vi "Main FPGA 5-axis with 1AxisLimitU8.vi"() -> ()   [LabVIEW 2013]
uses:
  <vilib>/Motion/MotorControl/_s/nism.interpretControlRegister.stateTransition.ctl
  <vilib>/Platform/TimedLoop/XDataNode/timing_clust.ctl
  <vilib>/Platform/TimedLoop/XDataNode/nitl_modes.ctl
  <vilib>/Platform/TimedLoop/XDataNode/wakeup.ctl
  <vilib>/Motion/MotorControl/_s/nism.digitalInputs.portA.ctl
  <vilib>/rvi/Emulation/niFpgaSctlEmulationGetInTimedLoop.vi
  <vilib>/rvi/Emulation/niFpgaEmulationReportErrorSimple.vi
  <vilib>/rvi/Emulation/niFpgaGetClockAttributes.vi
  <vilib>/rvi/Emulation/niFpgaCriticalErrorInLSC.vi
  Global FPGA.vi
  <vilib>/rvi/eio/common/nirviEmuTemplateMethod_errors.vi
  <vilib>/Motion/SoftMotion/Synchronization/nism.rioScan.generateSyncScan.vi
  <vilib>/rvi/Emulation/niFpgaProcessEmulError.vi
  <vilib>/Motion/MotorControl/_s/nism.interpretControlRegister.indexed.vi
  <vilib>/Motion/MotorControl/_s/nism.generateStatusRegister.indexed.vi
  <vilib>/Motion/MotorControl/_s/nism.mdo.read.positionLoopSyncData.vi
  <vilib>/Motion/MotorControl/_s/nism.mdo.read.splineData.vi
  <vilib>/Motion/MotorControl/_s/nism.splineInterpolation.fxp.3.index.vi
  <vilib>/Motion/MotorControl/_s/nism.mdo.handler.indexed.vi
  <vilib>/Motion/MotorControl/_s/nism.interpretDIOControl.portA.single.2.vi
  <vilib>/Motion/MotorControl/_s/nism.generateDIOStatus.portA.single.vi
  <vilib>/Platform/TimedLoop/XDataNode/XDataNode.xnode
  <vilib>/eio/EIONode/EIONode.xnode
  <vilib>/Motion/MotorControl/NI_SoftMotion_MotorControlIP.lvlib
  <vilib>/Platform/TimedLoop/XDataNode/XDNodeRunTimeDep.lvlib
  <vilib>/Motion/SoftMotion/Synchronization/NI_SoftMotion_Synchronization.lvlib
panel:
  in  "Axi1 1 DI":u8
  out "Axis Positions":fxp<+/-,64,32>[](array[numeric])
  in  "STEP or CW? (T=STEP)":bool
  out "Drive Enable":bool[](array[boolean])
  in  "Enable Watchdog":bool
  in  "Pet Watchdog":bool
  in  "Watchdog Timeout Period (ticks)":u64=40000000 format="%.0p"
  out "Watchdog Timed Out?":bool
  out "Time Since Last Pet":u64
  in  "Enable value":bool
  in  "Drive Enable override?":bool
  out "State":T1=enum."Start --> Initializing" caption="state transition"
  in  "Sync Value":bool
  in  "Sync Enable override?":bool
  in  "Invert direction?":bool
  out "Sync is Fault":bool
  out "Sync is Locked":bool
  in  "minimum pulse":u16=40
  # "Synchronization Loop"
  # "Control Status Loop"
  # "Notes: \n1. This VI provides the communication interface between the NI SoftMotion Engine and the LabVIEW FPGA Module. You must compile this VI for a specific FPGA target before use. After compiling, run the VI before running any of the Express VI examples. For information on moving this example to another FPGA target, refer to ni.com/info and enter info code fpgaex.\n\n2. Only use the Reset Axis button if you are unable to communicate with the axis by any other means. This button resets the device state machine and other VIs to a known state. After resetting the axis, switch the NI Scan Engine from Active Mode to Configuration Mode, then back to Active Mode, before attempting to enable the axis."
  # "(These two buttons \nare for testing\npurposes.)"
  # "(These two buttons \nare for testing\npurposes.)"
  # "Step/Direction Loop"
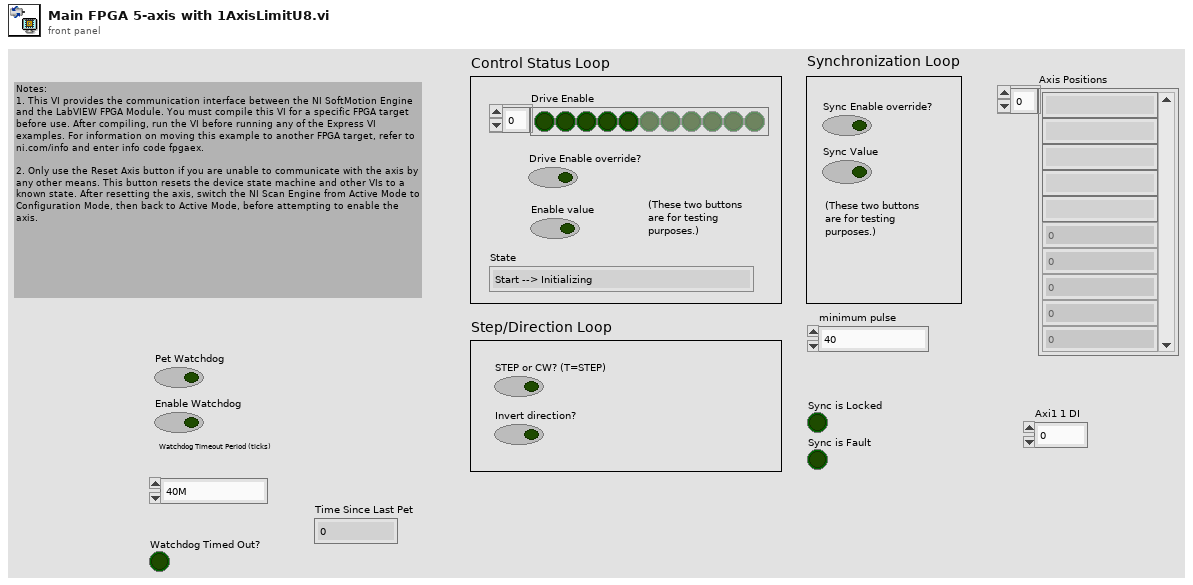
[diagram p1: front panel]
types:
  T1 = typedef "NI_SoftMotion_MotorControlIP.lvlib/nism.interpretControlRegister.stateTransition.ctl" = enum8{"Invalid", "Start --> Initializing", "Initializing --> Disabled", "Disabled --> Ready To Switch On", "Ready To Switch On --> Switched On", "Ready To Switch On --> Disable", "Switched On --> Operation Enable", "Switched On --> Ready To Switch On", "Switched On --> Disabled", "Operation Enable --> Switched On", "Operation Enable --> Ready To Switch On", "Operation Enable --> Disabled", "Fault --> Disabled", "Any --> Fault", "None"}
  T2 = typedef "NI_SoftMotion_MotorControlIP.lvlib/nism.mdo.splineData.ctl" = cluster{"spline type":T3, "traj per/spline per":u16, "spline per/traj per":fxp<+,32,0>}
  T3 = typedef "nism.splineInterpolation.type.ctl" = u16
  T4 = typedef "NI_SoftMotion_Synchronization.lvlib/nism.softmotionScan.timerConfig.ctl" = cluster{"Target Period (clocks)":u16, "Host Period / Target Period":u16}
  T5 = typedef "XDNodeRunTimeDep.lvlib/timing_clust.ctl" = cluster{"Expected End [f-1]":u64, "Actual End [f-1]":u64, "Finished Late? [f-1]":bool, "Expected End [i-1]":u64, "Actual End [i-1]":u64, "Finished Late? [i-1]":bool, "Expected Start [i]":u64, "Actual Start [i]":u64, "Expected Start [f]":u64, "Actual Start [f]":u64, "Source Name":string, "Structure Name":string, "Period":i64, "Deadline":i64, "Offset":i64, "Start":i64, "Priority":i32, "Timeout":i32, "Mode":T6, "Wakeup Reason":T7, "Error":errorcluster, "Source Type":string, "Secondary Source Type":string, "Global End Time":u64, "Global Start Time":u64, "Frame Duration":u64, "Iteration Duration":u64, "Assigned CPU":i32, "I/O Scan Engine Mode":u32}
  T6 = typedef "XDNodeRunTimeDep.lvlib/nitl_modes.ctl" = enum32{"No Change", "Process missed periods, maintain original phase", "Discard missed periods, maintain original phase", "Process missed periods, ignore original phase", "Discard missed periods, ignore original phase"}
  T7 = typedef "XDNodeRunTimeDep.lvlib/wakeup.ctl" = enum32{"Normal", "Aborted", "Asynchronous wakeup", "Timing source error", "Timed loop error", "Timeout"}
  T8 = typedef "NI_SoftMotion_Synchronization.lvlib/nism.softmotionScan.timerControl.ctl" = cluster{"SM Scan":bool, "SM Scan Count":u32, "SM Scan Enabled":bool}
  T9 = typedef "NI_SoftMotion_MotorControlIP.lvlib/nism.digitalInputs.portA.ctl" = cluster{"reverse limit":bool, "forward limit":bool, "home switch":bool, "digital input 0":bool, "digital input 1":bool, "digital input 2":bool, "digital input 3":bool}
  T10 = typedef "NI_SoftMotion_MotorControlIP.lvlib/nism.dio.portA.config.2.ctl" = cluster{"digital filter (us)":u16[], "safe state":enum16{"Low", "High", "No Change"}[]}
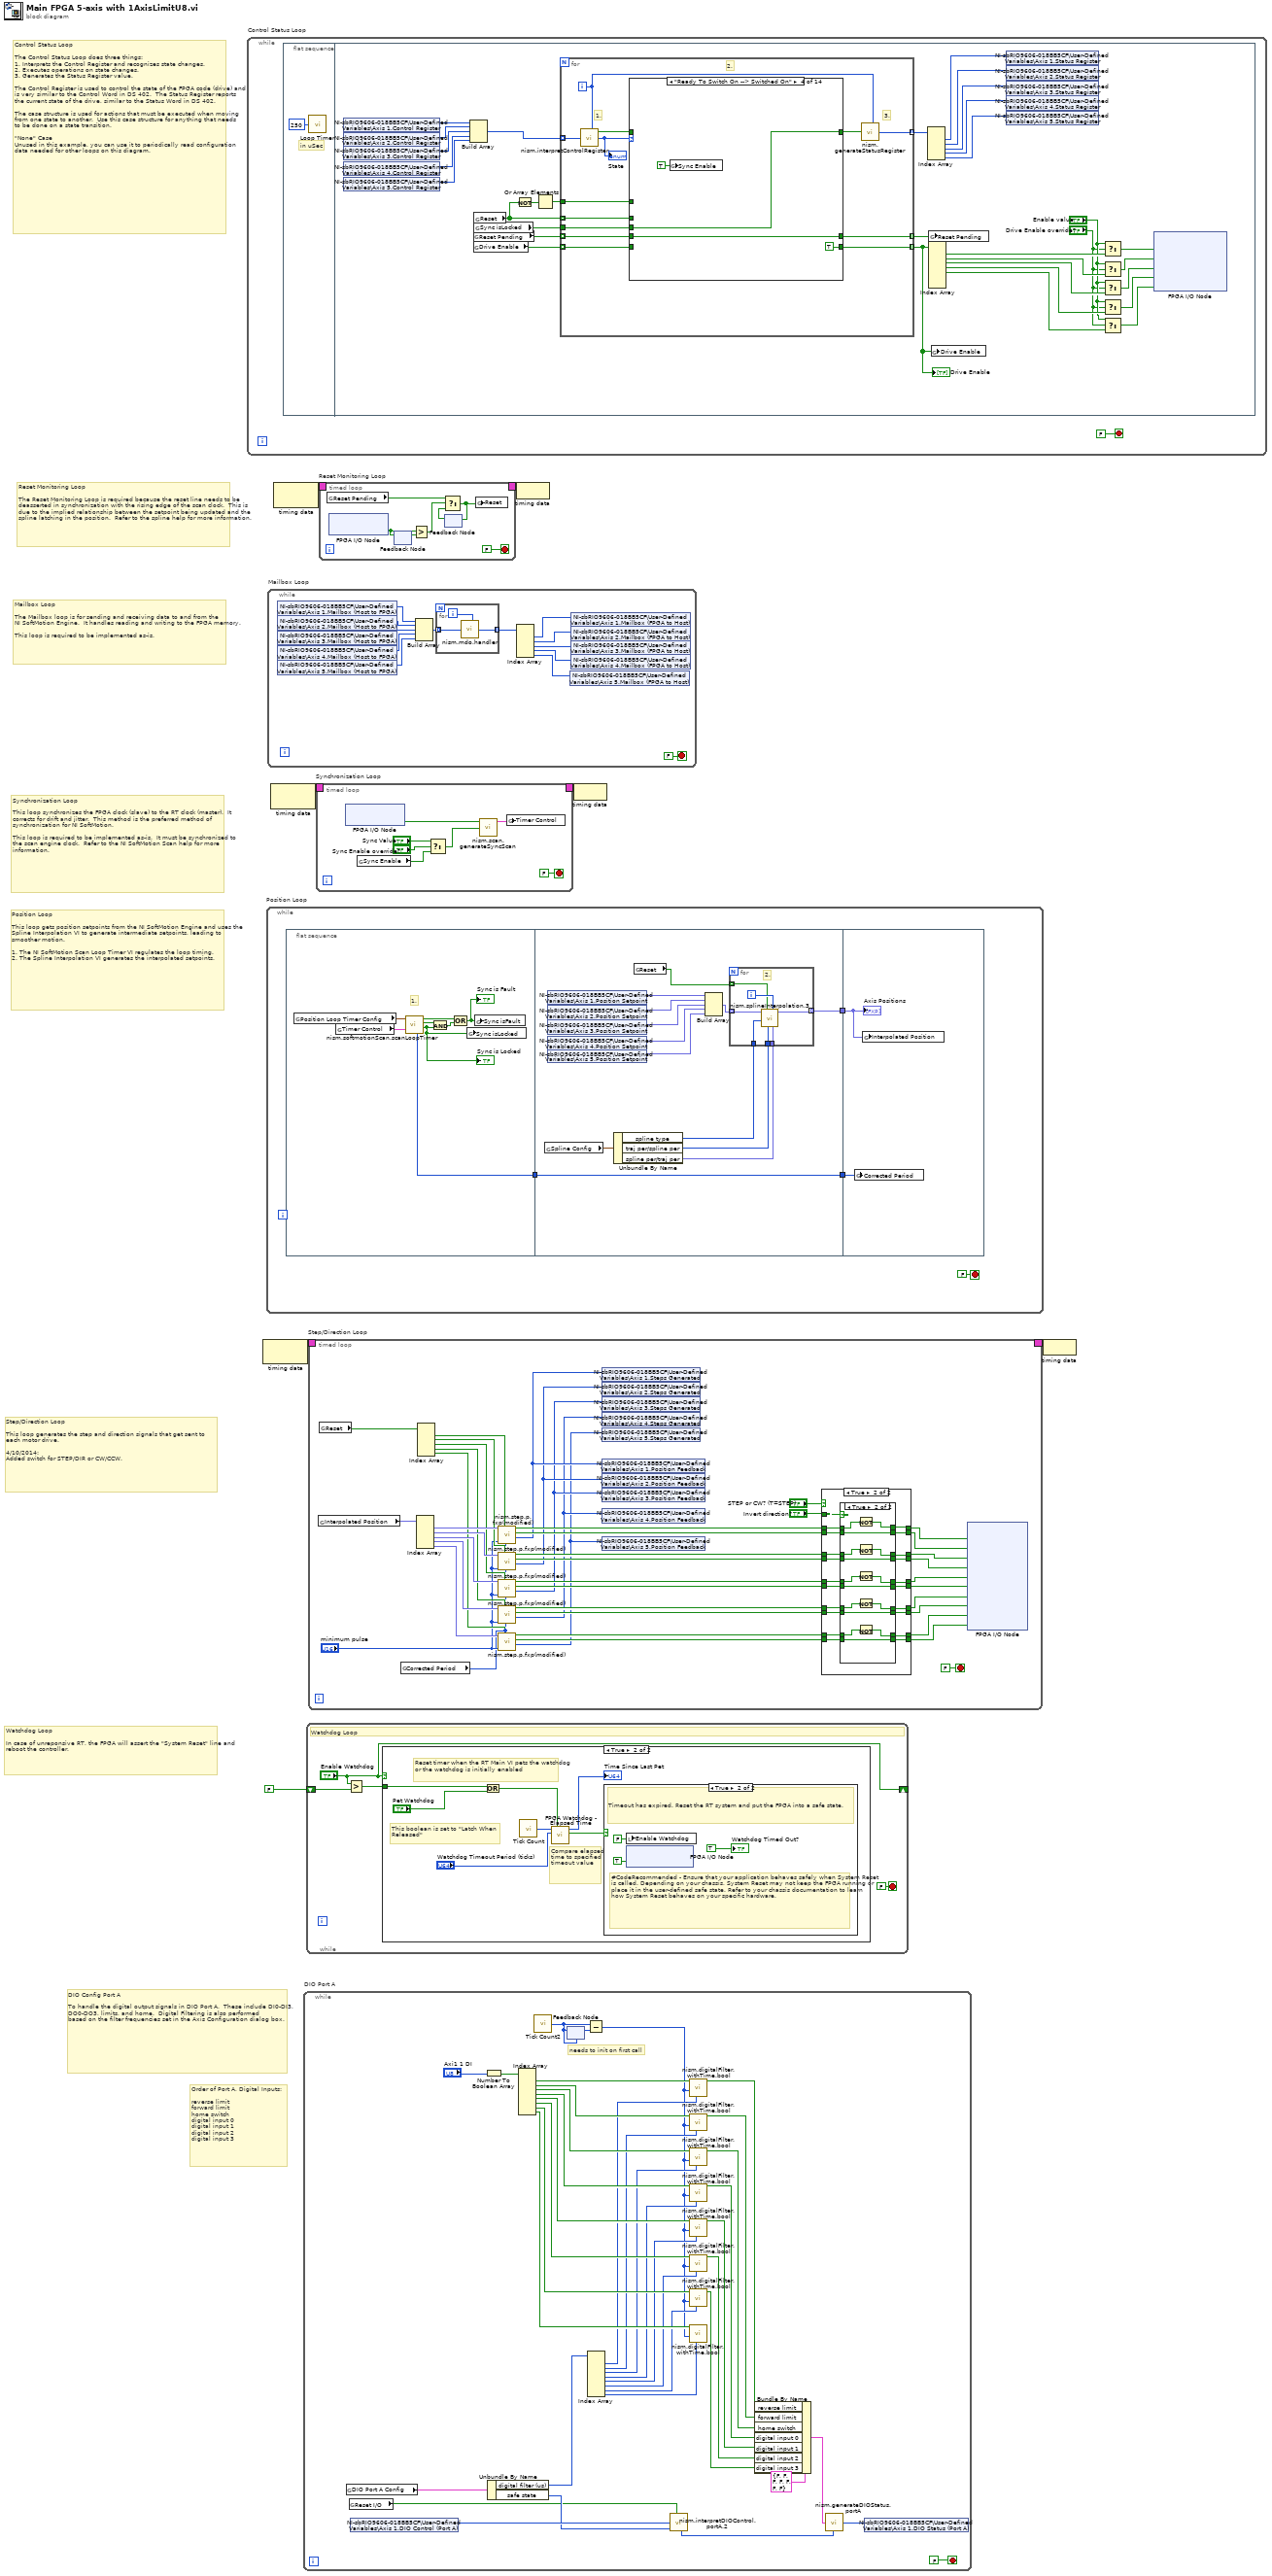
[diagram p0: block diagram]
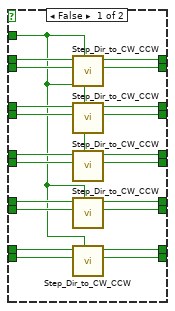
[diagram p4: hidden frame]
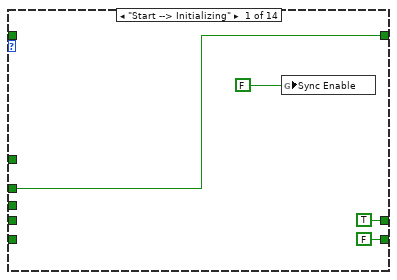
[diagram p6: hidden frame]
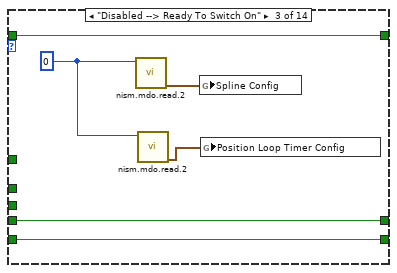
[diagram p8: hidden frame]
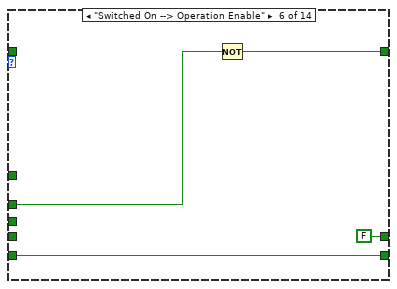
[diagram p10: hidden frame]
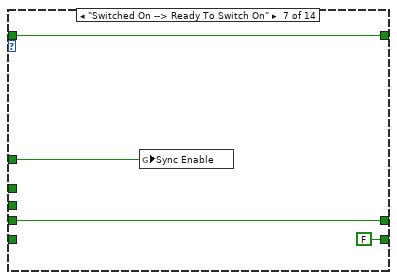
[diagram p11: hidden frame]
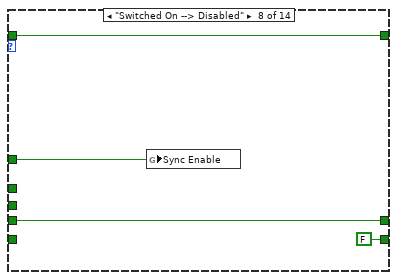
[diagram p12: hidden frame]
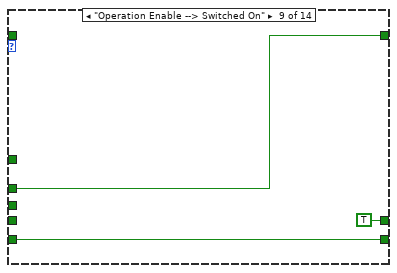
[diagram p13: hidden frame]
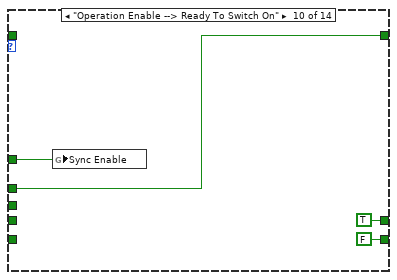
[diagram p14: hidden frame]
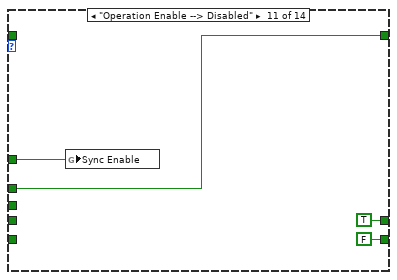
[diagram p15: hidden frame]
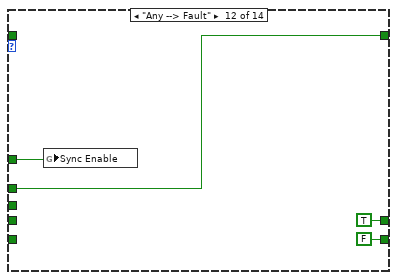
[diagram p16: hidden frame]
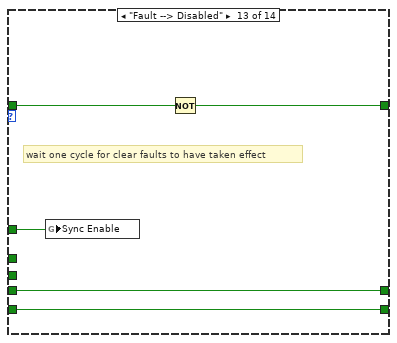
[diagram p17: hidden frame]
diagram:
  # "DIO Config Port A\n\nTo handle the digital output signals in DIO Port A.  These include DI0-DI3, DO0-DO3, limits, and home.  Digital Filtering is also performed\nbased on the filter frequencies set in the Axis Configuration dialog box."
  # "Order of Port A, Digital Inputs:\n\nreverse limit\nforward limit\nhome switch\ndigital input 0\ndigital input 1\ndigital input 2\ndigital input 3"
  # "Watchdog Loop\n\nIn case of unreponsive RT, the FPGA will assert the \"System Reset\" line and reboot the controller."
  # "Step/Direction Loop\n\nThis loop generates the step and direction signals that get sent to \neach motor drive.\n\n4/10/2014:\nAdded switch for STEP/DIR or CW/CCW."
  # "Position Loop\n\nThis loop gets position setpoints from the NI SoftMotion Engine and uses the Spline Interpolation VI to generate intermediate setpoints, leading to smoother motion.\n\n1. The NI SoftMotion Scan Loop Timer VI regulates the loop timing. \n2. The Spline Interpolation VI generates the interpolated setpoints."
  # "Synchronization Loop\n\nThis loop synchronizes the FPGA clock (slave) to the RT clock (master).  It corrects for drift and jitter.  This method is the preferred method of synchronization for NI SoftMotion.\n\nThis loop is required to be implemented as-is.  It must be synchronized to the scan engine clock.  Refer to the NI SoftMotion Scan help for more information."
  # "Mailbox Loop\n\nThe Mailbox loop is for sending and receiving data to and from the \nNI SoftMotion Engine.  It handles reading and writing to the FPGA memory.\n\nThis loop is required to be implemented as-is."
  # "Reset Monitoring Loop\n\nThe Reset Monitoring Loop is required because the reset line needs to be deasserted in synchronization with the rising edge of the scan clock.  This is due to the implied relationship between the setpoint being updated and the spline latching in the position.  Refer to the spline help for more information."
  # "Control Status Loop\n\nThe Control Status Loop does three things:\n1. Interprets the Control Register and recognizes state changes.\n2. Executes operations on state changes.\n3. Generates the Status Register value.\n\nThe Control Register is used to control the state of the FPGA code (drive) and is very similar to the Control Word in DS 402.  The Status Register reports the current state of the drive, similar to the Status Word in DS 402.\n\nThe case structure is used for actions that must be executed when moving from one state to another.  Use this case structure for anything that needs to be done on a state transition.\n\n\"None\" Case\nUnused in this example, you can use it to periodically read configuration data needed for other loops on this diagram."
  n1 = while "Control Status Loop" {
    stop <- FALSE stop-if-true
    n2 = flat-sequence {
      frame #0 {
        # "in uSec"
        n3 = call "Loop Timer"("Count(uSec)"=u32 250) -> ()  [unwired: 1 out]
      }
      frame #1 {
        n4 = shared-variable "NI-sbRIO9606-018BB5CF\\User-Defined Variables\\Axis 1.Control Register"() -> (w31:u32)  [unwired: 1 in, 1 out]
        n5 = shared-variable "NI-sbRIO9606-018BB5CF\\User-Defined Variables\\Axis 2.Control Register"() -> (w30:u32)  [unwired: 1 in, 1 out]
        n6 = shared-variable "NI-sbRIO9606-018BB5CF\\User-Defined Variables\\Axis 3.Control Register"() -> (w29:u32)  [unwired: 1 in, 1 out]
        n7 = shared-variable "NI-sbRIO9606-018BB5CF\\User-Defined Variables\\Axis 4.Control Register"() -> (w28:u32)  [unwired: 1 in, 1 out]
        n8 = shared-variable "NI-sbRIO9606-018BB5CF\\User-Defined Variables\\Axis 5.Control Register"() -> (w27:u32)  [unwired: 1 in, 1 out]
        n9 = Build Array(w31, w30, w29, w28, w27) -> (w40:u32[])
        n10 = global read "Global FPGA.vi" "Reset Pending"() -> (w35:bool[])
        n11 = global read "Global FPGA.vi" "Drive Enable"() -> (w34:bool[])
        n12 = global read "Global FPGA.vi" "Reset"() -> (w36:bool[])
        n13 = global read "Global FPGA.vi" "Sync isLocked"() -> (w41:bool)
        n14 = Not(x=w36) -> (.not. x?=w38:bool[])
        n15 = Or Array Elements(Boolean array=w38) -> (logical OR=w37:bool)
        n16 = for {
          tunnel: w36 -> [w49] mode=indexing
          tunnel: w41 -> [w48]
          tunnel: w40 -> [w50] mode=indexing
          tunnel: [w47] -> w32 mode=indexing
          tunnel: [w46] -> w39 mode=indexing
          tunnel: [w45] -> w33 mode=indexing
          tunnel: w37 -> [w44]
          tunnel: w35 -> [w43] mode=indexing
          tunnel: w34 -> [w42] mode=indexing
          i -> [w51]
          # "3."
          # "2."
          # "1."
          n17 = call-poly <vilib>:"nism.interpretControlRegister.vi"("control register"=w50, "axis index"=w51) -> ("transition occurred"=w52:bool, "state transition"=w53:T1)  [unwired: 6 in]
          "State" <- w53
          n18 = case shown="\"Ready To Switch On --> Switched On\"" w53 {
            tunnel: w52 -> [_ w61 w67 _ w74 _ w82 w86 _ _ _ _ w106 _]
            tunnel: [w58 w61 w67 w69 w74 w78 w82 w86 w88 w91 w95 w99 w105 _] -> w54
            tunnel: w49 -> [w58 _ _ _ _ w77 _ _ w88 w91 w95 w99 _ _]
            tunnel: w48 -> [_ _ _ w69 _ _ _ _ _ _ _ _ _ _]
            tunnel: [TRUE ("Write.Reset Pending") w60 w63 w68 w73 FALSE ("Write.Reset Pending") w79 w83 TRUE ("Write.Reset Pending") TRUE ("Write.Reset Pending") TRUE ("Write.Reset Pending") TRUE ("Write.Reset Pending") w103 w108] -> w46
            tunnel: [FALSE ("Write.Drive Enable") w59 w62 TRUE ("Write.Drive Enable") w72 w75 FALSE ("Write.Drive Enable") FALSE ("Write.Drive Enable") w87 FALSE ("Write.Drive Enable") FALSE ("Write.Drive Enable") FALSE ("Write.Drive Enable") w102 w107] -> w45
            tunnel: w44 -> [_ _ _ _ _ _ w80 w84 _ w90 w94 w98 w104 _]
            tunnel: w43 -> [_ w60 w63 w68 w73 _ w79 w83 _ _ _ _ w103 w108]
            tunnel: w42 -> [_ w59 w62 _ w72 w75 _ _ w87 _ _ _ w102 w107]
            frame "Start --> Initializing" {
              n19 = global write "Global FPGA.vi" "Sync Enable"(FALSE ("Sync Enable")) -> ()
            }
            frame "Initializing --> Disabled" {
            }
            frame "Disabled --> Ready To Switch On" {
              w65 = 0 ("axis index")
              n20 = call-poly <vilib>:"nism.mdo.read.2.vi"("axis index"=w65) -> ("spline"=w66:T2)  [unwired: 10 in]
              n21 = call-poly <vilib>:"nism.mdo.read.2.vi"("axis index"=w65) -> ("position loop sync"=w64:T4)  [unwired: 10 in]
              n22 = global write "Global FPGA.vi" "Spline Config"(w66) -> ()
              n23 = global write "Global FPGA.vi" "Position Loop Timer Config"(w64) -> ()
            }
            frame "Ready To Switch On --> Switched On" {
              n24 = global write "Global FPGA.vi" "Sync Enable"(TRUE ("Sync Enable")) -> ()
            }
            frame "Ready To Switch On --> Disable" {
            }
            frame "Switched On --> Operation Enable" {
              n25 = Not(x=w77) -> (.not. x?=w78:bool)
            }
            frame "Switched On --> Ready To Switch On" {
              n26 = global write "Global FPGA.vi" "Sync Enable"(w80) -> ()
            }
            frame "Switched On --> Disabled" {
              n27 = global write "Global FPGA.vi" "Sync Enable"(w84) -> ()
            }
            frame "Operation Enable --> Switched On" {
            }
            frame "Operation Enable --> Ready To Switch On" {
              n28 = global write "Global FPGA.vi" "Sync Enable"(w90) -> ()
            }
            frame "Operation Enable --> Disabled" {
              n29 = global write "Global FPGA.vi" "Sync Enable"(w94) -> ()
            }
            frame "Any --> Fault" {
              n30 = global write "Global FPGA.vi" "Sync Enable"(w98) -> ()
            }
            frame "Fault --> Disabled" {
              # "wait one cycle for clear faults to have taken effect"
              n31 = global write "Global FPGA.vi" "Sync Enable"(w104) -> ()
              n32 = Not(x=w106) -> (.not. x?=w105:bool)
            }
            frame "None", Default {
            }
          }
          n33 = call-poly <vilib>:"nism.generateStatusRegister.vi"("transition success"=w54, "axis index"=w51) -> ("status register"=w47:u32)  [unwired: 7 in]
        }
        "Drive Enable" <- w33
        n34 = Index Array(array=w32) -> (element #1=w26:u32, element #2=w25:u32, element #3=w24:u32, element #4=w23:u32, element #5=w22:u32)  [unwired: 5 in]
        n35 = global write "Global FPGA.vi" "Reset Pending"(w39) -> ()
        n36 = Index Array(array=w33) -> (element #1=w21:bool, element #2=w19:bool, element #3=w17:bool, element #4=w15:bool, element #5=w13:bool)  [unwired: 8 in, 3 out]
        n37 = global write "Global FPGA.vi" "Drive Enable"(w33) -> ()
        n38 = shared-variable "NI-sbRIO9606-018BB5CF\\User-Defined Variables\\Axis 1.Status Register"(w26) -> ()  [unwired: 1 in, 1 out]
        n39 = shared-variable "NI-sbRIO9606-018BB5CF\\User-Defined Variables\\Axis 2.Status Register"(w25) -> ()  [unwired: 1 in, 1 out]
        n40 = shared-variable "NI-sbRIO9606-018BB5CF\\User-Defined Variables\\Axis 3.Status Register"(w24) -> ()  [unwired: 1 in, 1 out]
        n41 = shared-variable "NI-sbRIO9606-018BB5CF\\User-Defined Variables\\Axis 4.Status Register"(w23) -> ()  [unwired: 1 in, 1 out]
        n42 = shared-variable "NI-sbRIO9606-018BB5CF\\User-Defined Variables\\Axis 5.Status Register"(w22) -> ()  [unwired: 1 in, 1 out]
        n43 = Select(t="Enable value", s="Drive Enable override?", f=w21) -> (s? t:f=w20:bool)
        n44 = Select(t="Enable value", s="Drive Enable override?", f=w19) -> (s? t:f=w18:bool)
        n45 = Select(t="Enable value", s="Drive Enable override?", f=w17) -> (s? t:f=w16:bool)
        n46 = Select(t="Enable value", s="Drive Enable override?", f=w15) -> (s? t:f=w14:bool)
        n47 = Select(t="Enable value", s="Drive Enable override?", f=w13) -> (s? t:f=w12:bool)
        n48 = xnode "FPGA I/O Node"("Axis1_Servo On"=w20, "Axis2_Servo On"=w18, "Axis3_Servo On"=w16, "Axis4_Servo On"=w14, "Axis5_Servo On"=w12) -> ()  [unwired: 5 in, 5 out]
      }
    }
  }
  n49 = node-c288() -> (w7:T5)  [unwired: 1 in]
  n50 = while "Position Loop" {
    stop <- FALSE stop-if-true
    n51 = flat-sequence {
      tunnel: [w113] -> w109
      tunnel: [w127] -> w111
      tunnel: [w126] -> w110
      tunnel: w109 -> [w126]
      tunnel: w111 -> [w141]
      tunnel: w110 -> [w142]
      frame #0 {
        # "1."
        n52 = global read "Global FPGA.vi" "Position Loop Timer Config"() -> (w115:T4)
        n53 = global read "Global FPGA.vi" "Timer Control"() -> (w114:T8)
        n54 = call <vilib>:"nism.softmotionScan.scanLoopTimer.vi"("Timer Control"=w114, "Timer Config"=w115) -> ("Scan Running?"=w117:bool, "Finished Late?"=w119:bool, "Fault Occurred?"=w120:bool, "Corrected Period"=w113:u16)  [unwired: 5 in, 1 out]
        "Sync is Locked" <- w117
        n55 = Compound Arithmetic op=AND(w119, w117) -> (w118:bool)
        n56 = Compound Arithmetic op=OR(w120, w118) -> (w116:bool)
        "Sync is Fault" <- w116
        n57 = global write "Global FPGA.vi" "Sync isLocked"(w117) -> ()
        n58 = global write "Global FPGA.vi" "Sync isFault"(w116) -> ()
      }
      frame #1 {
        n59 = global read "Global FPGA.vi" "Spline Config"() -> (w129:T2)
        n60 = shared-variable "NI-sbRIO9606-018BB5CF\\User-Defined Variables\\Axis 1.Position Setpoint"() -> (w125:fxp<+/-,64,32>)  [unwired: 1 in, 1 out]
        n61 = shared-variable "NI-sbRIO9606-018BB5CF\\User-Defined Variables\\Axis 2.Position Setpoint"() -> (w124:fxp<+/-,64,32>)  [unwired: 1 in, 1 out]
        n62 = shared-variable "NI-sbRIO9606-018BB5CF\\User-Defined Variables\\Axis 3.Position Setpoint"() -> (w123:fxp<+/-,64,32>)  [unwired: 1 in, 1 out]
        n63 = shared-variable "NI-sbRIO9606-018BB5CF\\User-Defined Variables\\Axis 4.Position Setpoint"() -> (w122:fxp<+/-,64,32>)  [unwired: 1 in, 1 out]
        n64 = shared-variable "NI-sbRIO9606-018BB5CF\\User-Defined Variables\\Axis 5.Position Setpoint"() -> (w121:fxp<+/-,64,32>)  [unwired: 1 in, 1 out]
        n65 = Unbundle By Name(w129) -> ("spline type"=w133:T3, "traj per/spline per"=w132:u16, "spline per/traj per"=w131:fxp<+,32,0>)
        n66 = global read "Global FPGA.vi" "Reset"() -> (w128:bool[])
        n67 = Build Array(w125, w124, w123, w122, w121) -> (w130:fxp<+/-,64,32>[])
        n68 = for {
          tunnel: w133 -> [w140]
          tunnel: w132 -> [w139]
          tunnel: w131 -> [w138]
          tunnel: w128 -> [w135] mode=indexing
          tunnel: w130 -> [w137] mode=indexing
          tunnel: [w134] -> w127 mode=indexing
          i -> [w136]
          # "2."
          n69 = call-poly <vilib>:"nism.splineInterpolation.3.vi"("1 / calls per sample"=w138, "index"=w136, "calls per sample"=w139, "reset"=w135, "spline type"=w140, "x"=w137) -> ("xi"=w134:fxp<+/-,64,32>)  [unwired: 5 in]
        }
      }
      frame #2 {
        n70 = global write "Global FPGA.vi" "Corrected Period"(w142) -> ()
        n71 = global write "Global FPGA.vi" "Interpolated Position"(w141) -> ()
        "Axis Positions" <- w141
      }
    }
  }
  n72 = while "Mailbox Loop" {
    stop <- FALSE stop-if-true
    n73 = shared-variable "NI-sbRIO9606-018BB5CF\\User-Defined Variables\\Axis 1.Mailbox (Host to FPGA)"() -> (w152:u64)  [unwired: 1 in, 1 out]
    n74 = shared-variable "NI-sbRIO9606-018BB5CF\\User-Defined Variables\\Axis 2.Mailbox (Host to FPGA)"() -> (w151:u64)  [unwired: 1 in, 1 out]
    n75 = shared-variable "NI-sbRIO9606-018BB5CF\\User-Defined Variables\\Axis 3.Mailbox (Host to FPGA)"() -> (w150:u64)  [unwired: 1 in, 1 out]
    n76 = shared-variable "NI-sbRIO9606-018BB5CF\\User-Defined Variables\\Axis 4.Mailbox (Host to FPGA)"() -> (w149:u64)  [unwired: 1 in, 1 out]
    n77 = shared-variable "NI-sbRIO9606-018BB5CF\\User-Defined Variables\\Axis 5.Mailbox (Host to FPGA)"() -> (w148:u64)  [unwired: 1 in, 1 out]
    n78 = Build Array(w152, w151, w150, w149, w148) -> (w154:u64[])
    n79 = for {
      tunnel: w154 -> [w158] mode=indexing
      tunnel: [w157] -> w153 mode=indexing
      i -> [w156]
      n80 = call-poly <vilib>:"nism.mdo.handler.vi"("mbox (host to fpga)"=w158, "axis index"=w156) -> ("mbox (fpga to host)"=w157:u64)  [unwired: 7 in]
    }
    n81 = Index Array(array=w153) -> (element #1=w147:u64, element #2=w146:u64, element #3=w145:u64, element #4=w144:u64, element #5=w143:u64)  [unwired: 5 in]
    n82 = shared-variable "NI-sbRIO9606-018BB5CF\\User-Defined Variables\\Axis 5.Mailbox (FPGA to Host)"(w143) -> ()  [unwired: 1 in, 1 out]
    n83 = shared-variable "NI-sbRIO9606-018BB5CF\\User-Defined Variables\\Axis 1.Mailbox (FPGA to Host)"(w147) -> ()  [unwired: 1 in, 1 out]
    n84 = shared-variable "NI-sbRIO9606-018BB5CF\\User-Defined Variables\\Axis 2.Mailbox (FPGA to Host)"(w146) -> ()  [unwired: 1 in, 1 out]
    n85 = shared-variable "NI-sbRIO9606-018BB5CF\\User-Defined Variables\\Axis 3.Mailbox (FPGA to Host)"(w145) -> ()  [unwired: 1 in, 1 out]
    n86 = shared-variable "NI-sbRIO9606-018BB5CF\\User-Defined Variables\\Axis 4.Mailbox (FPGA to Host)"(w144) -> ()  [unwired: 1 in, 1 out]
  }
  n87 = node-c288() -> (w5:T5)  [unwired: 1 in]
  n88 = node-c288() -> (w3:T5)  [unwired: 1 in]
  n89 = while "DIO Port A" {
    stop <- FALSE stop-if-true
    # "needs to init on first call"
    n90 = global read "Global FPGA.vi" "DIO Port A Config"() -> (w190:T10)
    n91 = global read "Global FPGA.vi" "Reset I/O"() -> (w188:bool)
    n92 = shared-variable "NI-sbRIO9606-018BB5CF\\User-Defined Variables\\Axis 1.DIO Control (Port A)"() -> (w194:u32)  [unwired: 1 in, 1 out]
    n93 = Number To Boolean Array(number="Axi1 1 DI") -> (Boolean array=w187:bool[])
    n94 = Unbundle By Name(w190) -> ("digital filter (us)"=w167:u16[], "safe state"=w189:enum16{"Low", "High", "No Change"}[])
    n95 = Index Array(array=w187) -> (element #1=w186:bool, element #2=w179:bool, element #3=w180:bool, element #4=w181:bool, element #5=w182:bool, element #6=w183:bool, element #7=w184:bool, element #8=w185:bool)  [unwired: 8 in]
    n96 = call "Tick Count2"() -> ("Tick Count(uSec)"=w169:u16)
    n97 = feedback #1(w169) -> (w170:u16)
    n98 = feedback-in #1(w169) -> ()
    n99 = Subtract(x=w169, y=w170) -> (x-y=w168:u16)
    n100 = Index Array(array=w167) -> (element #1=w171:u16, element #2=w172:u16, element #3=w173:u16, element #4=w174:u16, element #5=w175:u16, element #6=w176:u16, element #7=w177:u16, element #8=w178:u16)  [unwired: 8 in]
    n101 = call-poly <vilib>:"nism.interpretDIOControl.portA.2.vi"("reset"=w188, "dio control(port a)"=w194, "safe state"=w189) -> ("reset latches"=w196:u8)  [unwired: 5 in, 1 out]
    n102 = call <vilib>:"nism.digitalFilter.withTime.bool.vi"("filter value"=w171, "delta time"=w168, "input signal"=w186) -> ("output signal"=w166:bool)  [unwired: 8 in]
    n103 = call <vilib>:"nism.digitalFilter.withTime.bool.vi"("filter value"=w172, "delta time"=w168, "input signal"=w179) -> ("output signal"=w165:bool)  [unwired: 8 in]
    n104 = call <vilib>:"nism.digitalFilter.withTime.bool.vi"("filter value"=w173, "delta time"=w168, "input signal"=w180) -> ("output signal"=w164:bool)  [unwired: 8 in]
    n105 = call <vilib>:"nism.digitalFilter.withTime.bool.vi"("filter value"=w174, "delta time"=w168, "input signal"=w181) -> ("output signal"=w163:bool)  [unwired: 8 in]
    n106 = call <vilib>:"nism.digitalFilter.withTime.bool.vi"("filter value"=w175, "delta time"=w168, "input signal"=w182) -> ("output signal"=w162:bool)  [unwired: 8 in]
    n107 = call <vilib>:"nism.digitalFilter.withTime.bool.vi"("filter value"=w176, "delta time"=w168, "input signal"=w183) -> ("output signal"=w161:bool)  [unwired: 8 in]
    n108 = call <vilib>:"nism.digitalFilter.withTime.bool.vi"("filter value"=w177, "delta time"=w168, "input signal"=w184) -> ("output signal"=w160:bool)  [unwired: 8 in]
    n109 = call <vilib>:"nism.digitalFilter.withTime.bool.vi"("filter value"=w178, "delta time"=w168, "input signal"=w185) -> ()  [unwired: 8 in, 1 out]
    n110 = Bundle By Name(cluster=T9 {"reverse limit"=FALSE, "forward limit"=FALSE, "home switch"=FALSE, "digital input 0"=FALSE, "digital input 1"=FALSE, "digital input 2"=FALSE, "digital input 3"=FALSE} ("$(driveInterface.digitalInputs.shortName)"), "reverse limit"=w166, "forward limit"=w165, "home switch"=w164, "digital input 0"=w163, "digital input 1"=w162, "digital input 2"=w161, "digital input 3"=w160) -> (w192:T9)
    n111 = call-poly <vilib>:"nism.generateDIOStatus.portA.vi"("digital inputs"=w192, "reset latches"=w196) -> ("dio status(port a)"=w195:u32)  [unwired: 7 in]
    n112 = shared-variable "NI-sbRIO9606-018BB5CF\\User-Defined Variables\\Axis 1.DIO Status (Port A)"(w195) -> ()  [unwired: 1 in, 1 out]
  }
  n113 = while "RT Watchdog Loop" {
    shift-right: ["Enable Watchdog"] -> _
    shift-left: FALSE ("Enable RT Watchdog") -> [w200]
    stop <- FALSE stop-if-true
    # "Watchdog Loop"
    n114 = Greater?(x="Enable Watchdog", y=w200) -> (0:w197:bool)
    n115 = case shown="True" "Enable Watchdog" {
      tunnel: w197 -> [_ w203]
      frame False {
        # "This loop has to be explicitly enabled from the RT Main VI.  This reduces the possiblity of an endless reboot cycle."
      }
      frame True {
        # "This boolean is set to \"Latch When Released\""
        # "Compare elapsed time to specified timeout value"
        # "Reset timer when the RT Main VI pets the watchdog or the watchdog is initially enabled"
        n116 = Or(x=w203, y="Pet Watchdog") -> (x .or. y?=w202:bool)
        n117 = call "Tick Count"() -> ("Tick Count(Ticks)"=w206:u32)
        n118 = call "FPGA Watchdog - Elapsed Time.vi"("Reset"=w202, "Timeout Period"="Watchdog Timeout Period (ticks)", "Current Time"=w206) -> ("Timeout"=w201:bool, "Elapsed Time"=→"Time Since Last Pet":u64)  [unwired: 7 in]
        n119 = case shown="True" w201 {
          frame False {
            # "Timeout has not expired."
          }
          frame True {
            # "#CodeRecommended - Ensure that your application behaves safely when System Reset is called. Depending on your chassis, System Reset may not keep the FPGA running or place it in the user-defined safe state. Refer to your chassis documentation to learn how System Reset behaves on your specific hardware."
            # "Timeout has expired. Reset the RT system and put the FPGA into a safe state."
            n120 = local write "Enable Watchdog"(FALSE ("Enable RT Watchdog")) -> ()
            n121 = xnode "FPGA I/O Node"("System Reset"=TRUE ("RT Reset on Watchdog Failure?")) -> ()  [unwired: 1 in, 1 out]
            "Watchdog Timed Out?" <- TRUE ("Watchdog Timed Out?")
          }
        }
      }
    }
  }
  n122 = timed-loop "Step/Direction Loop" {
    timing: w7 -> [_]
    timing-out: [_] -> w6
    stop <- FALSE stop-if-true
    n123 = global read "Global FPGA.vi" "Interpolated Position"() -> (w251:fxp<+/-,64,32>[])
    n124 = global read "Global FPGA.vi" "Reset"() -> (w245:bool[])
    n125 = global read "Global FPGA.vi" "Corrected Period"() -> (w211:u16)
    n126 = Index Array(array=w251) -> (element #1=w250:fxp<+/-,64,32>, element #2=w249:fxp<+/-,64,32>, element #3=w248:fxp<+/-,64,32>, element #4=w247:fxp<+/-,64,32>, element #5=w246:fxp<+/-,64,32>)  [unwired: 5 in]
    n127 = Index Array(array=w245) -> (element #1=w244:bool, element #2=w243:bool, element #3=w242:bool, element #4=w241:bool, element #5=w240:bool)  [unwired: 5 in]
    n128 = call "nism.step.p.fxp(modified).vi"("calls per sample"=w211, "reset"=w244, "minimum pulse"="minimum pulse", "position setpoint"=w250) -> ("steps generated"=w216:i32, "step"=w238:bool, "direction"=w239:bool)  [unwired: 4 in, 1 out]
    n129 = call "nism.step.p.fxp(modified).vi"("calls per sample"=w211, "reset"=w243, "minimum pulse"="minimum pulse", "position setpoint"=w249) -> ("steps generated"=w215:i32, "step"=w236:bool, "direction"=w237:bool)  [unwired: 4 in, 1 out]
    n130 = call "nism.step.p.fxp(modified).vi"("calls per sample"=w211, "reset"=w242, "minimum pulse"="minimum pulse", "position setpoint"=w248) -> ("steps generated"=w214:i32, "step"=w234:bool, "direction"=w235:bool)  [unwired: 4 in, 1 out]
    n131 = call "nism.step.p.fxp(modified).vi"("calls per sample"=w211, "reset"=w241, "minimum pulse"="minimum pulse", "position setpoint"=w247) -> ("steps generated"=w213:i32, "step"=w232:bool, "direction"=w233:bool)  [unwired: 4 in, 1 out]
    n132 = call "nism.step.p.fxp(modified).vi"("calls per sample"=w211, "reset"=w240, "minimum pulse"="minimum pulse", "position setpoint"=w246) -> ("steps generated"=w212:i32, "step"=w230:bool, "direction"=w231:bool)  [unwired: 4 in, 1 out]
    n133 = shared-variable "NI-sbRIO9606-018BB5CF\\User-Defined Variables\\Axis 1.Steps Generated"(w216) -> ()  [unwired: 1 in, 1 out]
    n134 = shared-variable "NI-sbRIO9606-018BB5CF\\User-Defined Variables\\Axis 2.Steps Generated"(w215) -> ()  [unwired: 1 in, 1 out]
    n135 = shared-variable "NI-sbRIO9606-018BB5CF\\User-Defined Variables\\Axis 3.Steps Generated"(w214) -> ()  [unwired: 1 in, 1 out]
    n136 = shared-variable "NI-sbRIO9606-018BB5CF\\User-Defined Variables\\Axis 4.Steps Generated"(w213) -> ()  [unwired: 1 in, 1 out]
    n137 = shared-variable "NI-sbRIO9606-018BB5CF\\User-Defined Variables\\Axis 5.Steps Generated"(w212) -> ()  [unwired: 1 in, 1 out]
    n138 = shared-variable "NI-sbRIO9606-018BB5CF\\User-Defined Variables\\Axis 1.Position Feedback"(w216) -> ()  [unwired: 1 in, 1 out]
    n139 = shared-variable "NI-sbRIO9606-018BB5CF\\User-Defined Variables\\Axis 2.Position Feedback"(w215) -> ()  [unwired: 1 in, 1 out]
    n140 = shared-variable "NI-sbRIO9606-018BB5CF\\User-Defined Variables\\Axis 3.Position Feedback"(w214) -> ()  [unwired: 1 in, 1 out]
    n141 = shared-variable "NI-sbRIO9606-018BB5CF\\User-Defined Variables\\Axis 4.Position Feedback"(w213) -> ()  [unwired: 1 in, 1 out]
    n142 = shared-variable "NI-sbRIO9606-018BB5CF\\User-Defined Variables\\Axis 5.Position Feedback"(w212) -> ()  [unwired: 1 in, 1 out]
    n143 = case shown="True" "STEP or CW? (T=STEP)" {
      tunnel: w239 -> [w273 w293]
      tunnel: w238 -> [w272 w283]
      tunnel: w237 -> [w271 w291]
      tunnel: w236 -> [w270 w281]
      tunnel: w235 -> [w269 w289]
      tunnel: w234 -> [w268 w279]
      tunnel: w233 -> [w267 w287]
      tunnel: w232 -> [w266 w277]
      tunnel: w231 -> [w265 w285]
      tunnel: w230 -> [w264 w275]
      tunnel: "Invert direction?" -> [w253 w294]
      tunnel: [w263 w292] -> w228
      tunnel: [w262 w282] -> w219
      tunnel: [w261 w290] -> w227
      tunnel: [w260 w280] -> w226
      tunnel: [w259 w288] -> w225
      tunnel: [w258 w278] -> w224
      tunnel: [w257 w286] -> w223
      tunnel: [w256 w276] -> w222
      tunnel: [w255 w284] -> w221
      tunnel: [w254 w274] -> w220
      frame False {
        n144 = call "Step_Dir_to_CW_CCW.vi"("invert"=w253, "step"=w272, "direction"=w273) -> ("CCW"=w262:bool, "CW"=w263:bool)  [unwired: 7 in]
        n145 = call "Step_Dir_to_CW_CCW.vi"("invert"=w253, "step"=w270, "direction"=w271) -> ("CCW"=w260:bool, "CW"=w261:bool)  [unwired: 7 in]
        n146 = call "Step_Dir_to_CW_CCW.vi"("invert"=w253, "step"=w268, "direction"=w269) -> ("CCW"=w258:bool, "CW"=w259:bool)  [unwired: 7 in]
        n147 = call "Step_Dir_to_CW_CCW.vi"("invert"=w253, "step"=w266, "direction"=w267) -> ("CCW"=w256:bool, "CW"=w257:bool)  [unwired: 7 in]
        n148 = call "Step_Dir_to_CW_CCW.vi"("invert"=w253, "step"=w264, "direction"=w265) -> ("CCW"=w254:bool, "CW"=w255:bool)  [unwired: 7 in]
      }
      frame True {
        n149 = case shown="True" w294 {
          tunnel: w293 -> [w304 w319]
          tunnel: [w304 w318] -> w292
          tunnel: w291 -> [w302 w317]
          tunnel: [w302 w316] -> w290
          tunnel: w289 -> [w300 w315]
          tunnel: [w300 w314] -> w288
          tunnel: w287 -> [w298 w313]
          tunnel: [w298 w312] -> w286
          tunnel: w285 -> [w296 w311]
          tunnel: [w296 w310] -> w284
          tunnel: w283 -> [w303 w309]
          tunnel: [w303 w309] -> w282
          tunnel: w281 -> [w301 w308]
          tunnel: [w301 w308] -> w280
          tunnel: w279 -> [w299 w307]
          tunnel: [w299 w307] -> w278
          tunnel: w277 -> [w297 w306]
          tunnel: [w297 w306] -> w276
          tunnel: w275 -> [w295 w305]
          tunnel: [w295 w305] -> w274
          frame False {
          }
          frame True {
            n150 = Not(x=w319) -> (.not. x?=w318:bool)
            n151 = Not(x=w317) -> (.not. x?=w316:bool)
            n152 = Not(x=w315) -> (.not. x?=w314:bool)
            n153 = Not(x=w313) -> (.not. x?=w312:bool)
            n154 = Not(x=w311) -> (.not. x?=w310:bool)
          }
        }
      }
    }
    n155 = xnode "FPGA I/O Node"("Axis1_CW"=w228, "Axis1_CCW"=w219, "Axis2_CW"=w227, "Axis2_CCW"=w226, "Axis3_CW"=w225, "Axis3_CCW"=w224, "Axis4_CW"=w223, "Axis4_CCW"=w222, "Axis5_CW"=w221, "Axis5_CCW"=w220) -> ()  [unwired: 10 in, 10 out]
  }
  n156 = timed-loop "Synchronization Loop" {
    timing: w5 -> [_]
    timing-out: [_] -> w4
    stop <- FALSE stop-if-true
    n157 = xnode "FPGA I/O Node"() -> ("Scan Clock"=w326:bool)  [unwired: 1 in, 1 out]
    n158 = global read "Global FPGA.vi" "Sync Enable"() -> (w325:bool)
    n159 = Select(t="Sync Value", s="Sync Enable override?", f=w325) -> (s? t:f=w322:bool)
    n160 = call-poly <vilib>:"nism.scan.generateSyncScan.vi"("Scan Enable?"=w322, "Scan Clock"=w326) -> ("Timer Control"=w327:T8)  [unwired: 3 in]
    n161 = global write "Global FPGA.vi" "Timer Control"(w327) -> ()
  }
  n162 = timed-loop "Reset Monitoring Loop" {
    timing: w3 -> [_]
    timing-out: [_] -> w2
    stop <- FALSE stop-if-true
    n163 = global read "Global FPGA.vi" "Reset Pending"() -> (w333:bool[])
    n164 = xnode "FPGA I/O Node"() -> ("Scan Clock"=w332:bool)  [unwired: 1 in, 1 out]
    n165 = feedback-in #2(w332) -> ()
    n166 = feedback #2() -> (w331:bool)  [unwired: 1 in]
    n167 = Greater?(x=w332, y=w331) -> (0:w337:bool)
    n168 = feedback #3() -> (w336:bool[])  [unwired: 1 in]
    n169 = Select(t=w333, s=w337, f=w336) -> (s? t:f=w334:bool[])
    n170 = feedback-in #3(w334) -> ()
    n171 = global write "Global FPGA.vi" "Reset"(w334) -> ()
  }
  n172 = node-c288(w2) -> ()
  n173 = node-c288(w4) -> ()
  n174 = node-c288(w6) -> ()
